vi "StartAttract.vi"(8 "error in (no error)":errorcluster, 10 "Start?":bool, 11 "Engine in":refnum<class "Engine.lvclass">) -> (0 "error out":errorcluster, 3 "Engine out":refnum<class "Engine.lvclass">)   [LabVIEW 2019, in "RT_Game.lvlib" / "Engine.lvclass"]
uses:
  Engine.lvclass
  Engine.lvclass/Engine.ctl
  AttractScreen/AttractScreen.lvclass
  C:/Users/FreshBob/Dropbox/VIs/myRIO_GameConsole/RT/RT_Game/Game/Game.lvclass
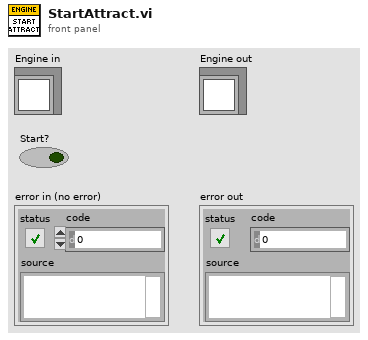
[diagram p1: front panel]
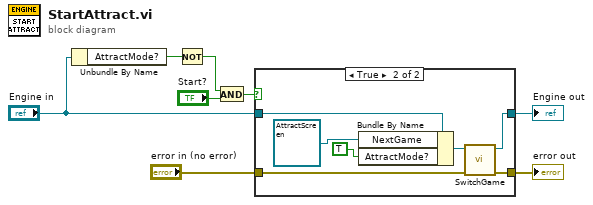
[diagram p0: block diagram]
diagram:
  n1 = Unbundle By Name("Engine in") -> ("AttractMode?"=w2:bool)
  n2 = Not(x=w2) -> (.not. x?=w1:bool)
  n3 = And(x=w1, y="Start?") -> (x .and. y?=w4:bool)
  n4 = case shown="True" w4 {
    tunnel: "error in (no error)" -> [w9 w17]
    tunnel: [w10 w14] -> w6
    tunnel: [w9 w16] -> w7
    tunnel: "Engine in" -> [w10 w15]
    frame False {
    }
    frame True {
      n5 = Bundle By Name(cluster=w15, "NextGame"=refnum<class "AttractScreen.lvclass"> refnum ("RT_Game.lvlib:AttractScreen.lvclass"), "AttractMode?"=TRUE) -> (w13:refnum<class "Engine.lvclass">)
      n6 = call "SwitchGame.vi"("error in (no error)"=w17, "Engine in"=w13) -> ("error out"=w16:errorcluster, "Engine out"=w14:refnum<class "Engine.lvclass">)  [unwired: 8 in]
    }
  }
  "error out" <- w7
  "Engine out" <- w6
